vi "Add Bus Controller.vi"(8 "error in":errorcluster, 11 "port in":T1 format="%.0x") -> (0 "error out":errorcluster, 2 "bus controller":T1 format="%.0x", 3 "port out":T1 format="%.0x")   [LabVIEW 2020, in "Ballard MIL-STD-1553 Scripting.lvlib"]
uses:
  Ballard MIL-STD-1553 Scripting.lvlib
  <vilib>/NI VeriStand/Custom Device API/Custom Device Item Ref.ctl
  <vilib>/NI VeriStand/Custom Device API/Custom Device Channel.ctl
  <vilib>/NI VeriStand/Custom Device API/Custom Device Channel Type.ctl
  Constants.vi
  <vilib>/NI VeriStand/Custom Device API/Custom Device API.lvlib
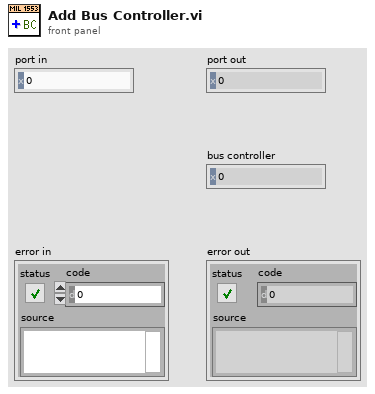
[diagram p1: front panel]
types:
  T1 = typedef "Custom Device API.lvlib/Custom Device Item Ref.ctl" = u64
  T2 = typedef "Custom Device API.lvlib/Custom Device Channel.ctl" = cluster{"Type":T3, "Units":string, "Default Value":dbl, "Faultable":bool, "Scalable":bool}
  T3 = typedef "Custom Device API.lvlib/Custom Device Channel Type.ctl" = enum16{"Input", "Output"}
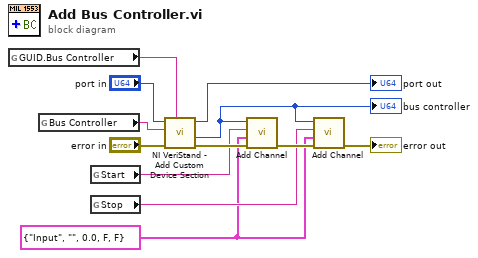
[diagram p0: block diagram]
diagram:
  w2 = T2 {"Type"=enum."Input", "Units"="", "Default Value"=0.0, "Faultable"=FALSE, "Scalable"=FALSE} ("Channel")
  n1 = global read "Constants.vi" "GUID.Bus Controller"() -> (w12:string)
  n2 = global read "Constants.vi" "Bus Controller"() -> (w8:string)
  n3 = global read "Constants.vi" "Start"() -> (w4:string)
  n4 = global read "Constants.vi" "Stop"() -> (w3:string)
  n5 = call <vilib>:"NI VeriStand - Add Custom Device Section.vi"("GUID (Default Section)"=w12, "error in (no error)"="error in", "Section Name"=w8, "Parent Ref in"="port in") -> ("error out"=w7:errorcluster, "Section Ptr"=w1:T1, "Parent Ref out"=→"port out":T1)  [unwired: 4 in, 1 out]
  "bus controller" <- w1
  n6 = call "Add Channel.vi"("error in"=w7, "Channel"=w2, "Name"=w4, "Frame Ref"=w1) -> ("error out"=w6:errorcluster)  [unwired: 6 in, 1 out]
  n7 = call "Add Channel.vi"("error in"=w6, "Channel"=w2, "Name"=w3, "Frame Ref"=w1) -> ("error out"=→"error out":errorcluster)  [unwired: 6 in, 1 out]
